vi "DAQ Manager.vi"(0 "DAQ Name":string="USB-6343", 1 "DAQ Mngr Action":T4, 9 "Value":dbl, 11 "error in (no error)":errorcluster) -> (3 "Vacuum Array":T1[](array[typedef]), 4 "device":tag, 6 "Pressure Array":T2[](array[typedef]), 8 "Plots":T3[](array[typedef]), 10 "Cart Sense":bool[](array[boolean]), 13 "Pressure Array":dbl[](array[numeric]), 14 "Connected":bool, 15 "error out":errorcluster)   [LabVIEW 2020]
uses:
  DAQ Mngr.ctl
  Main/Pressure Point.ctl
  Main/Pressure Output.ctl
  Main/Vacuum Output.ctl
  <vilib>/DAQmx/read.llb/DAQmx Read (Analog 2D DBL NChan NSamp).vi
  <vilib>/Analysis/baseanly.llb/Mean (DBL).vi
  <vilib>/DAQmx/write.llb/DAQmx Write (Digital 1D Bool 1Chan 1Samp).vi
  <vilib>/DAQmx/write.llb/DAQmx Write (Analog DBL 1Chan 1Samp).vi
  DAQ/DAQ Globals.vi
  <vilib>/DAQmx/miscellaneous.llb/DAQmx Fill In Error Info.vi
  <vilib>/DAQmx/create/channels.llb/DAQmx Create Channel (DO-Digital Output).vi
  <vilib>/DAQmx/create/channels.llb/DAQmx Create Channel (DI-Digital Input).vi
  <vilib>/DAQmx/create/channels.llb/DAQmx Create Channel (AO-Voltage-Basic).vi
  <vilib>/Analysis/NI_AALBase.lvlib
  Lib/Utilities.lvlib
panel:
  out "Vacuum Array":dbl[](array[numeric])
  in  "Buffer":u32=150
  out "PS Sense":bool
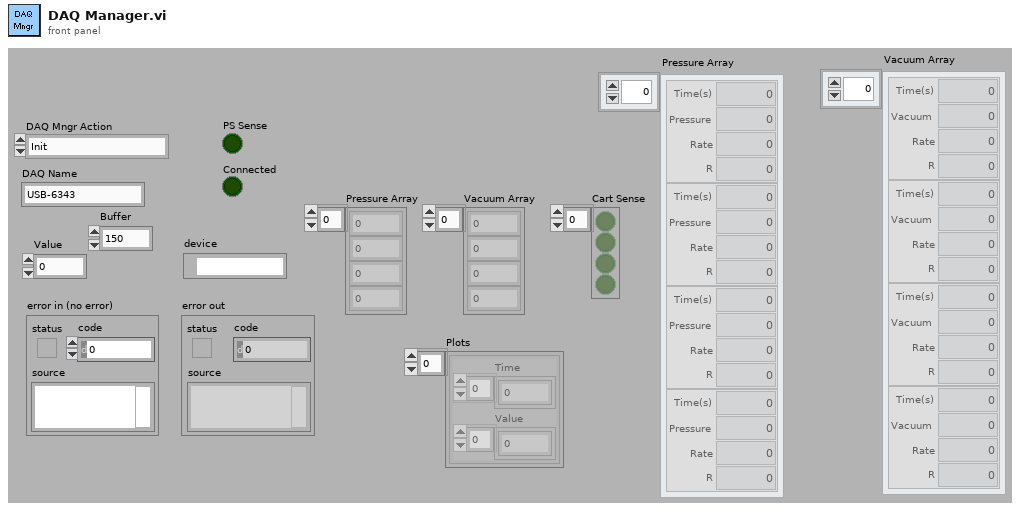
[diagram p1: front panel]
types:
  T1 = typedef "Vacuum Output.ctl" = cluster{"Time(s)":dbl, "Vacuum":dbl, "Rate":dbl, "R":dbl}
  T2 = typedef "Pressure Output.ctl" = cluster{"Time(s)":dbl, "Pressure":dbl, "Rate":dbl, "R":dbl}
  T3 = typedef "Pressure Point.ctl" = cluster{"Time":dbl[], "Value":dbl[]}
  T4 = typedef "DAQ Mngr.ctl" = enum16{"Init", "Read Pressure", "Read Vacuum", "Analyze Pressure", "Analyze Vacuum", "Read Cartridges", "Lock Cartridge", "Unlock Cartridge", "Read PS", "Pinch Valve Engage", "Pinch Valve Disengage", "Close"}
  T5 = cluster{"negative limit switch":bool, "positive limit switch":bool, "home switch":bool, "position marker":bool, "device enable":bool, "quick stop":bool, "general purpose J":bool, "general purpose I":bool, "general purpose H":bool, "general purpose G":bool, "general purpose F":bool, "general purpose E":bool, "general purpose D":bool, "general purpose C":bool, "general purpose B":bool, "general purpose A":bool}
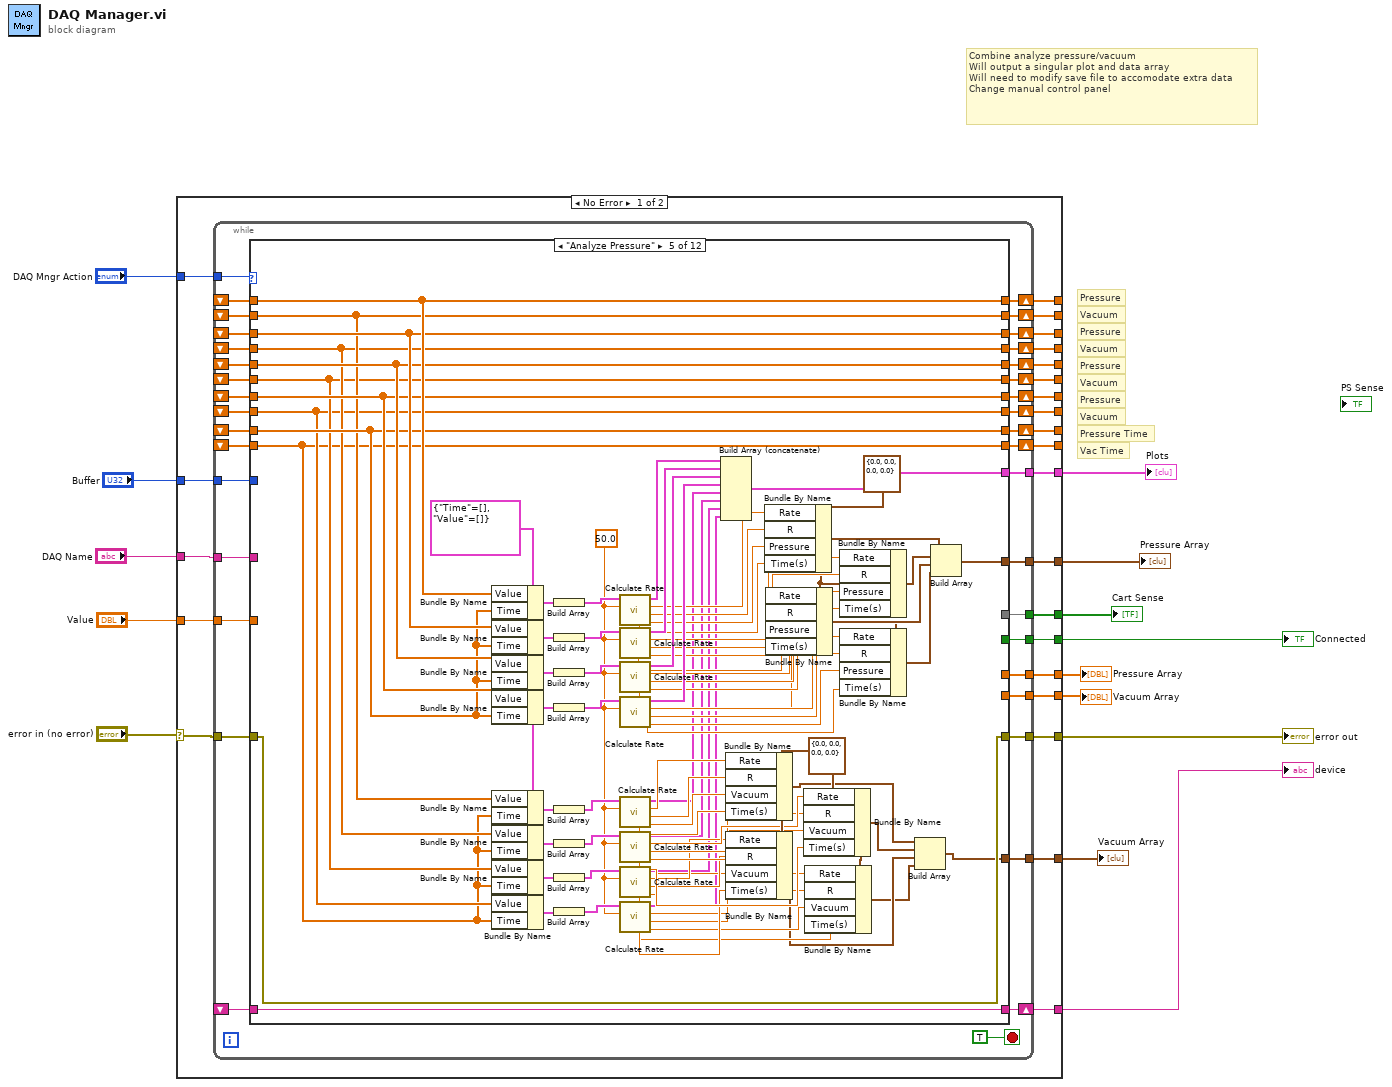
[diagram p0: block diagram]
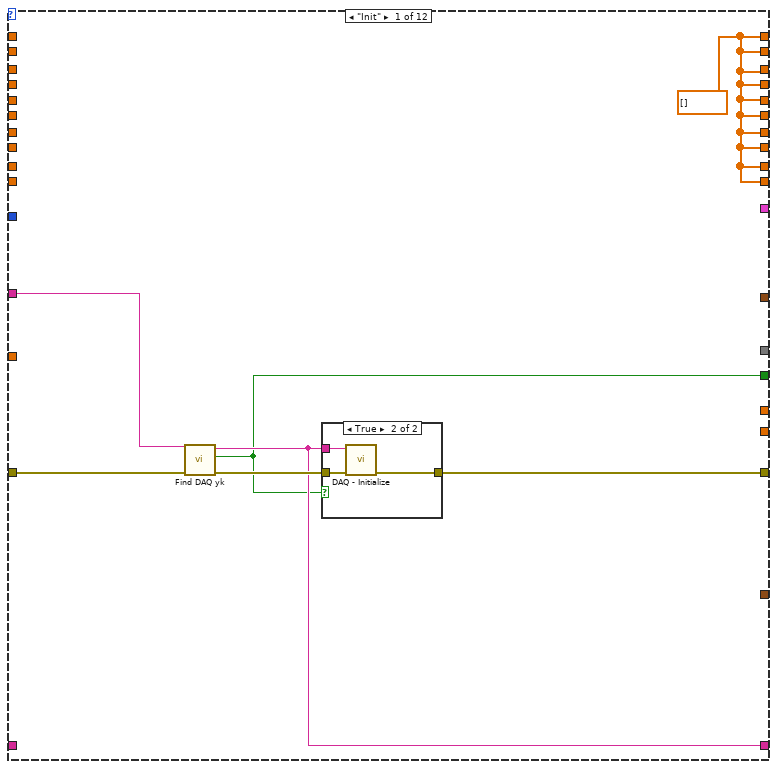
[diagram p2: hidden frame]
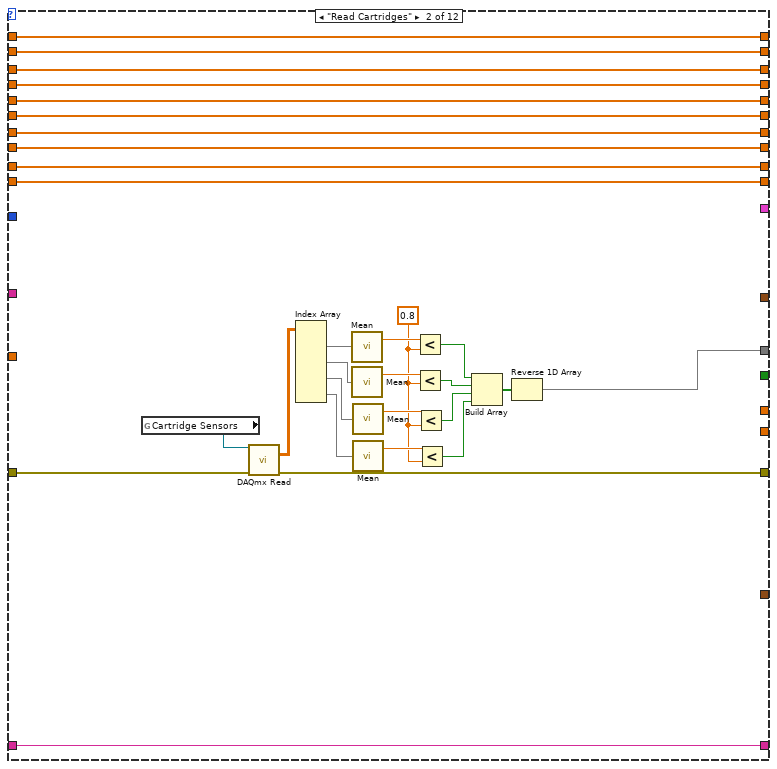
[diagram p4: hidden frame]
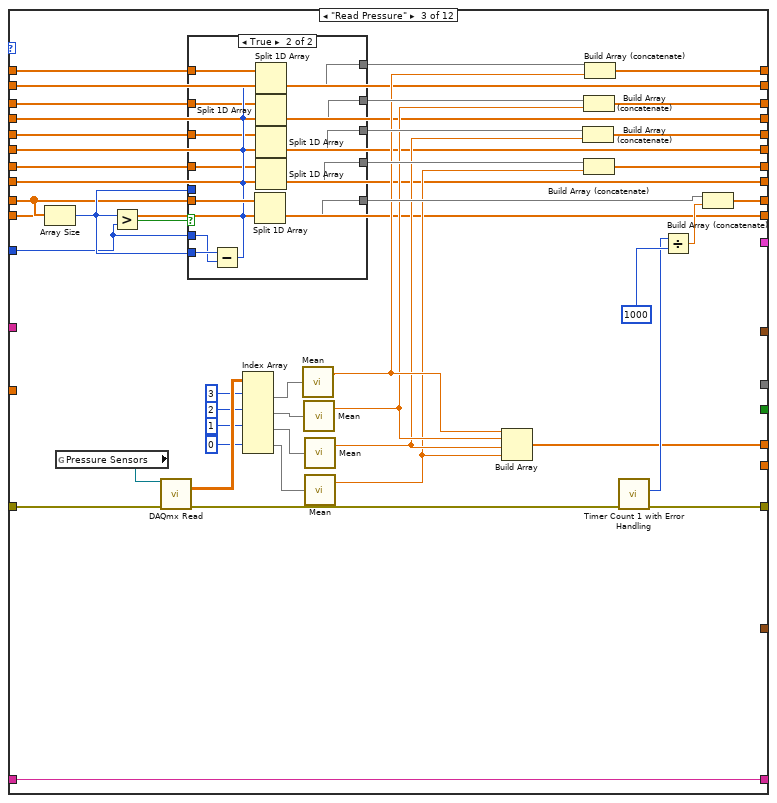
[diagram p5: hidden frame]
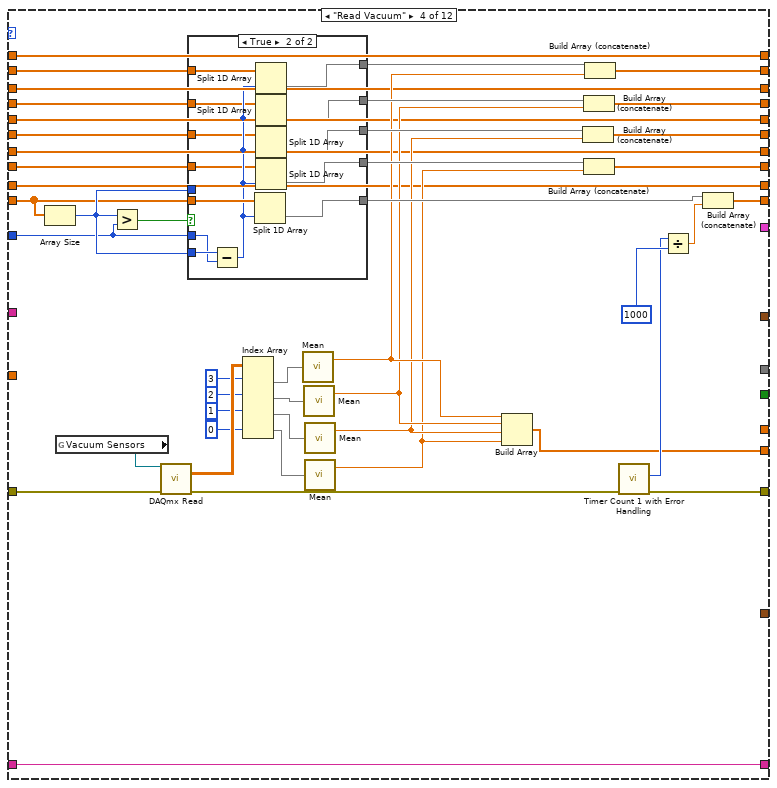
[diagram p7: hidden frame]
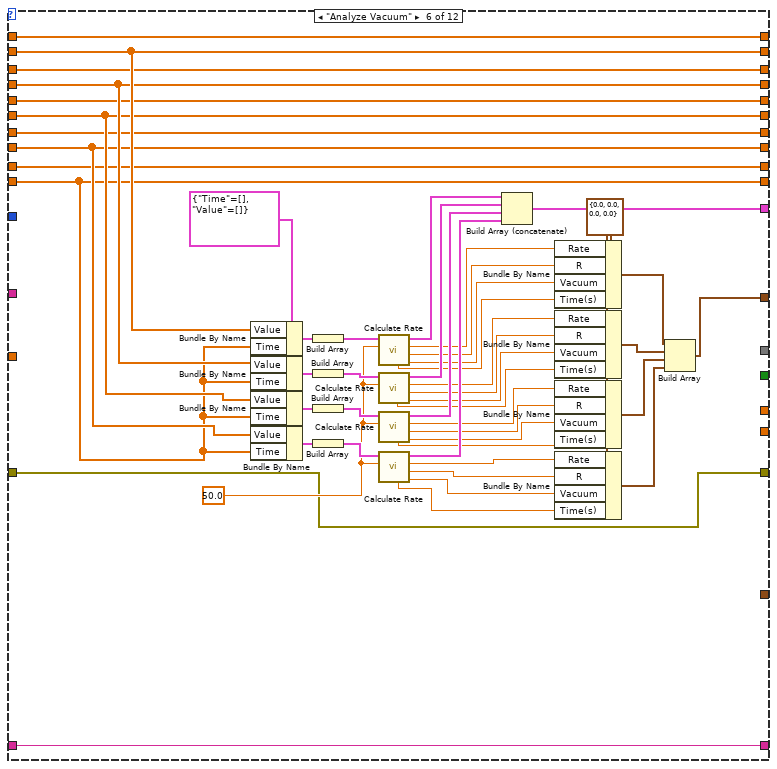
[diagram p9: hidden frame]
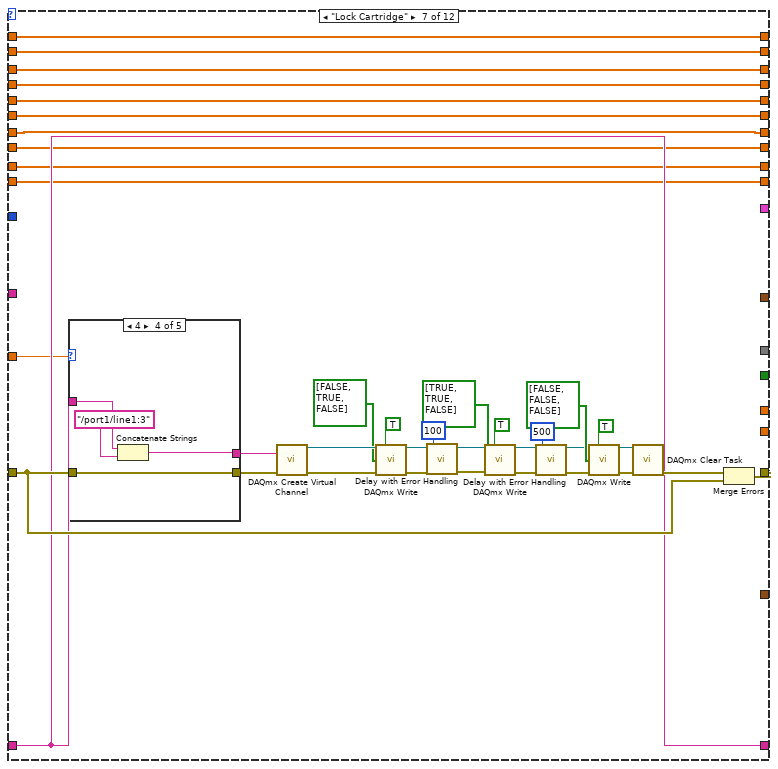
[diagram p10: hidden frame]
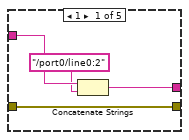
[diagram p11: hidden frame]
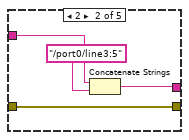
[diagram p12: hidden frame]
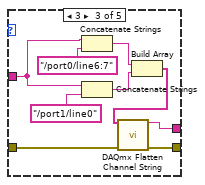
[diagram p13: hidden frame]
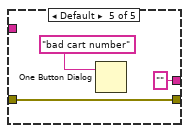
[diagram p14: hidden frame]
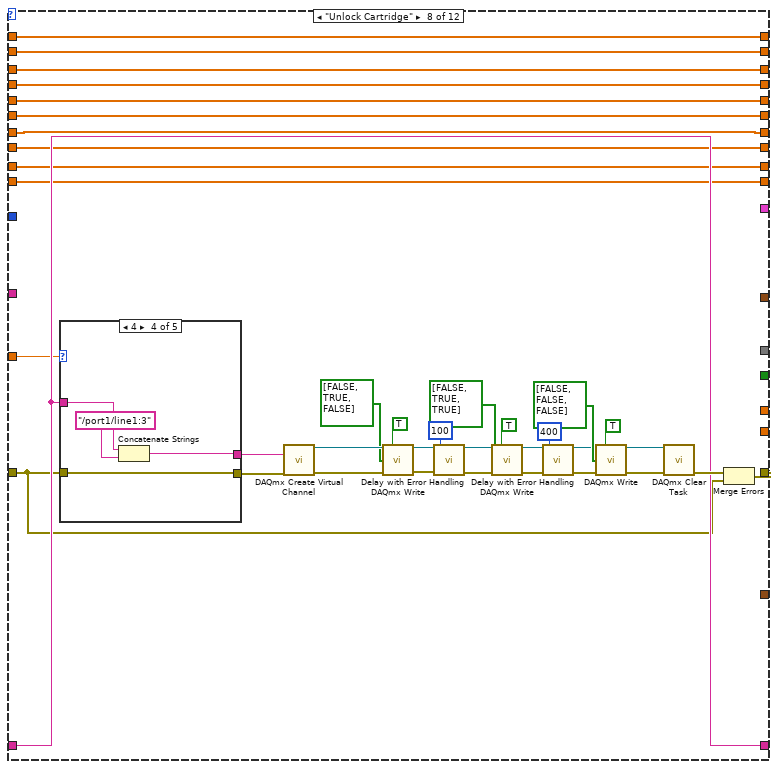
[diagram p15: hidden frame]
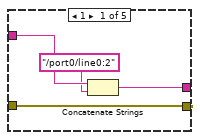
[diagram p16: hidden frame]
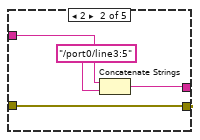
[diagram p17: hidden frame]
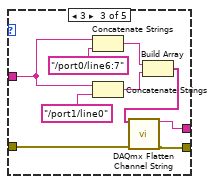
[diagram p18: hidden frame]
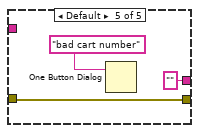
[diagram p19: hidden frame]
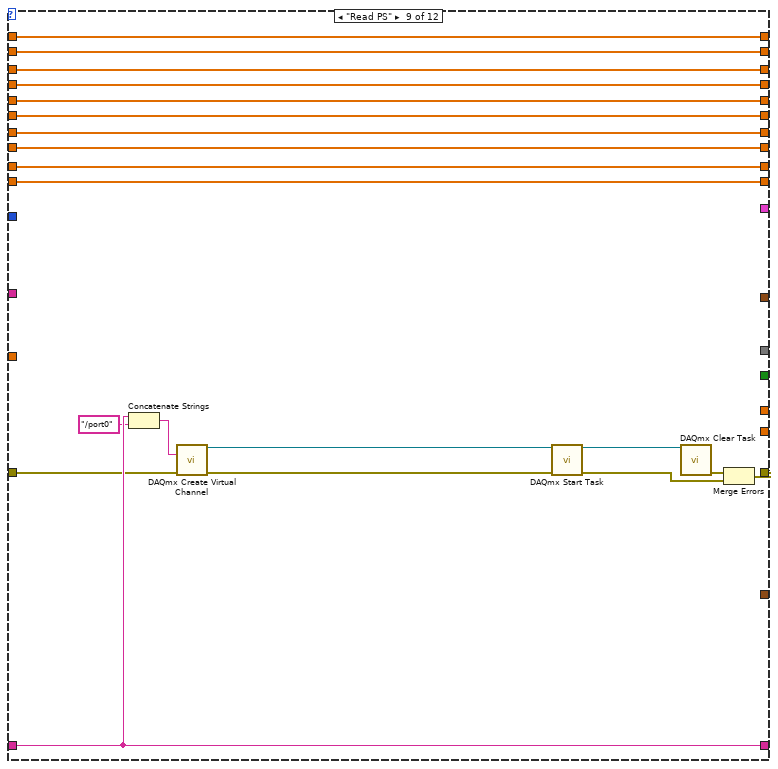
[diagram p20: hidden frame]
diagram:
  # "Vac Time"
  # "Pressure Time"
  # "Combine analyze pressure/vacuum\nWill output a singular plot and data array\nWill need to modify save file to accomodate extra data\nChange manual control panel"
  # "Vacuum"
  # "Pressure"
  # "Vacuum"
  # "Pressure"
  # "Vacuum"
  # "Pressure"
  # "Vacuum"
  # "Pressure"
  n1 = case shown="No Error" "error in (no error)" {
    selector: "error in (no error)" -> [w38 w616]
    tunnel: [w36 w616] -> w13
    tunnel: "DAQ Name" -> [w37 _]
    tunnel: "DAQ Mngr Action" -> [w35 _]
    tunnel: [w34 _] -> w10
    tunnel: [w33 _] -> w9
    tunnel: "Value" -> [w32 _]
    tunnel: [w31 _] -> w7
    tunnel: "Buffer" -> [w30 _]
    tunnel: [w29 _] -> _
    tunnel: [w28 _] -> _
    tunnel: [w27 _] -> _
    tunnel: [w26 _] -> _
    tunnel: [w25 _] -> _
    tunnel: [w24 _] -> w5
    tunnel: [w23 _] -> w3
    tunnel: [w22 _] -> w4
    tunnel: [w21 _] -> _
    tunnel: [w20 _] -> _
    tunnel: [w19 _] -> _
    tunnel: [w18 _] -> _
    tunnel: [w17 _] -> _
    tunnel: [w16 _] -> w2
    tunnel: [w15 _] -> w1
    frame No Error {
      n2 = while {
        tunnel: w38 -> [w72]
        tunnel: w37 -> [w71]
        tunnel: [w70] -> w36
        tunnel: w35 -> [w73]
        tunnel: [w69] -> w34
        tunnel: w32 -> [w67]
        shift-right: [w68] -> w33
        shift-left: _ -> [w66]
        tunnel: [w65] -> w31
        tunnel: w30 -> [w64]
        shift-right: [w63] -> w25
        shift-left: _ -> [w62]
        shift-right: [w61] -> w29
        shift-left: _ -> [w60]
        shift-right: [w59] -> w28
        shift-left: _ -> [w54]
        shift-right: [w58] -> w27
        shift-left: _ -> [w55]
        shift-right: [w57] -> w26
        shift-left: _ -> [w56]
        tunnel: [w53] -> w24
        tunnel: [w52] -> w23
        tunnel: [w51] -> w22
        shift-right: [w50] -> w21
        shift-left: _ -> [w45]
        shift-right: [w49] -> w20
        shift-left: _ -> [w44]
        shift-right: [w48] -> w19
        shift-left: _ -> [w43]
        shift-right: [w47] -> w18
        shift-left: _ -> [w42]
        shift-right: [w46] -> w17
        shift-left: _ -> [w41]
        tunnel: [w40] -> w16
        tunnel: [w39] -> w15
        stop <- TRUE stop-if-true
        n3 = case shown="\"Analyze Pressure\"" w73 {
          tunnel: w72 -> [w80 w114 w159 w222 w287 w340 w387 w464 w508 w551 w597 _]
          tunnel: w71 -> [w79 _ _ _ _ _ _ _ _ _ _ _]
          tunnel: [w78 w113 w142 w207 w287 w340 w407 w466 w509 w531 w577 w615] -> w70
          tunnel: [w76 _ _ _ _ _ _ _ _ _ _ _] -> w69
          tunnel: [w77 w115 w160 w223 w289 w343 w386 w465 w510 w519 w565 w609] -> w68
          tunnel: w67 -> [_ _ _ _ _ _ w385 w463 _ _ _ _]
          tunnel: w66 -> [_ w115 w160 w223 w289 w343 w386 w465 w510 w519 w565 w609]
          tunnel: [_ w96 _ _ _ _ _ _ _ _ _ _] -> w65
          tunnel: w64 -> [_ _ w145 w208 _ _ _ _ _ _ _ _]
          tunnel: [w75 w92 w144 w183 w321 w327 w380 w439 w498 w557 w603 w611] -> w63
          tunnel: w62 -> [_ w92 w143 w183 w321 w327 w380 w439 w498 w557 w603 w611]
          tunnel: [w75 w91 w140 w184 w320 w326 w379 w438 w497 w556 w602 w610] -> w61
          tunnel: w60 -> [_ w91 w139 w184 w320 w326 w379 w438 w497 w556 w602 w610]
          tunnel: [w75 w95 w138 w180 w324 w330 w383 w442 w501 w555 w601 w614] -> w59
          tunnel: [w75 w94 w137 w181 w323 w329 w382 w441 w500 w554 w600 w613] -> w58
          tunnel: [w75 w93 w136 w182 w322 w328 w381 w440 w499 w553 w599 w612] -> w57
          tunnel: w56 -> [_ w93 w135 w182 w322 w328 w381 w440 w499 w553 w599 w612]
          tunnel: w55 -> [_ w94 w134 w181 w323 w329 w382 w441 w500 w554 w600 w613]
          tunnel: w54 -> [_ w95 w133 w180 w324 w330 w383 w442 w501 w555 w601 w614]
          tunnel: [_ _ _ _ w319 w372 _ _ _ _ _ _] -> w53
          tunnel: [_ _ _ _ w291 w325 _ _ _ _ _ _] -> w52
          tunnel: [_ _ w125 _ _ _ _ _ _ _ _ _] -> w51
          tunnel: [w75 w90 w120 w194 w272 w336 w374 w437 w496 w516 w562 w608] -> w50
          tunnel: [w75 w89 w119 w193 w271 w335 w375 w436 w495 w515 w561 w607] -> w49
          tunnel: [w75 w88 w118 w192 w270 w334 w376 w435 w494 w514 w560 w606] -> w48
          tunnel: [w75 w87 w117 w191 w269 w333 w377 w434 w493 w513 w559 w605] -> w47
          tunnel: [w75 w86 w116 w190 w268 w332 w378 w433 w492 w512 w558 w604] -> w46
          tunnel: w45 -> [_ w90 w120 w189 w272 w336 w374 w437 w496 w516 w562 w608]
          tunnel: w44 -> [_ w89 w119 w188 w271 w335 w375 w436 w495 w515 w561 w607]
          tunnel: w43 -> [_ w88 w118 w187 w270 w334 w376 w435 w494 w514 w560 w606]
          tunnel: w42 -> [_ w87 w117 w186 w269 w333 w377 w434 w493 w513 w559 w605]
          tunnel: w41 -> [_ w86 w116 w185 w268 w332 w378 w433 w492 w512 w558 w604]
          tunnel: [_ _ _ w179 _ _ _ _ _ _ _ _] -> w40
          tunnel: [_ _ _ _ w246 _ _ _ _ _ _ _] -> w39
          frame "Init" {
            w75 = dbl[] []
            n4 = call "Find DAQ yk.vi"("error in"=w80, "DAQ Name"=w79) -> ("error out"=w81:errorcluster, "Device Found"=w76:bool, "device"=w77:tag)  [unwired: 5 in, 2 out]
            n5 = case shown="True" w76 {
              tunnel: w81 -> [w82 w85]
              tunnel: [w82 w84] -> w78
              tunnel: w77 -> [_ w83]
              frame False {
              }
              frame True {
                n6 = call "DAQ - Initialize.vi"("error in (no error)"=w85, "DAQ"=w83) -> ("error out"=w84:errorcluster)  [unwired: 9 in]
              }
            }
          }
          frame "Read Cartridges" {
            w102 = 0.8 ("y")
            n7 = global read "DAQ Globals.vi" "Cartridge Sensors"() -> (w112:refnum<k21>)
            n8 = call-poly <vilib>:"DAQmx Read.vi"("task/channels in"=w112, "error in"=w114) -> ("data"=w111:dbl[][], "error out"=w113:errorcluster)  [unwired: 11 in, 1 out]
            n9 = Index Array(array=w111) -> (element #1=w110:dbl[], element #2=w109:dbl[], element #3=w108:dbl[], element #4=w107:dbl[])  [unwired: 8 in]
            n10 = call-poly <vilib>:"Mean.vi"("X"=w110) -> ("mean"=w106:dbl)  [unwired: 1 out]
            n11 = call-poly <vilib>:"Mean.vi"("X"=w109) -> ("mean"=w105:dbl)  [unwired: 1 out]
            n12 = call-poly <vilib>:"Mean.vi"("X"=w108) -> ("mean"=w104:dbl)  [unwired: 1 out]
            n13 = call-poly <vilib>:"Mean.vi"("X"=w107) -> ("mean"=w103:dbl)  [unwired: 1 out]
            n14 = Less?(x=w106, y=w102) -> (x < y?=w101:bool)
            n15 = Less?(x=w105, y=w102) -> (x < y?=w100:bool)
            n16 = Less?(x=w104, y=w102) -> (x < y?=w99:bool)
            n17 = Less?(x=w103, y=w102) -> (x < y?=w98:bool)
            n18 = Build Array(w101, w100, w99, w98) -> (w97:bool[])
            n19 = Reverse 1D Array(array=w97) -> (reversed array=w96:bool[])
          }
          frame "Read Pressure" {
            n20 = Array Size(array=w139) -> (size(s)=w150:i32)
            n21 = global read "DAQ Globals.vi" "Pressure Sensors"() -> (w157:refnum<k21>)
            n22 = Greater?(x=w150, y=w145) -> (0:w151:bool)
            n23 = call-poly <vilib>:"DAQmx Read.vi"("task/channels in"=w157, "error in"=w159) -> ("data"=w156:dbl[][], "error out"=w158:errorcluster)  [unwired: 11 in, 1 out]
            n24 = case shown="True" w151 {
              tunnel: w143 -> [w165 w173]
              tunnel: w139 -> [w164 w178]
              tunnel: w145 -> [_ w176]
              tunnel: w150 -> [_ _]
              tunnel: w150 -> [_ w177]
              tunnel: [w165 w166] -> w149
              tunnel: [w164 w175] -> w148
              tunnel: w135 -> [w161 w172]
              tunnel: w134 -> [w162 w171]
              tunnel: w133 -> [w163 w170]
              tunnel: [w163 w169] -> w132
              tunnel: [w162 w168] -> w131
              tunnel: [w161 w167] -> w130
              frame False {
              }
              frame True {
                n25 = Subtract(x=w177, y=w176) -> (x-y=w174:u32)
                n26 = Split 1D Array(array=w178, index=w174) -> (second subarray=w175:dbl[])  [unwired: 1 out]
                n27 = Split 1D Array(array=w170, index=w174) -> (second subarray=w169:dbl[])  [unwired: 1 out]
                n28 = Split 1D Array(array=w171, index=w174) -> (second subarray=w168:dbl[])  [unwired: 1 out]
                n29 = Split 1D Array(array=w172, index=w174) -> (second subarray=w167:dbl[])  [unwired: 1 out]
                n30 = Split 1D Array(array=w173, index=w174) -> (second subarray=w166:dbl[])  [unwired: 1 out]
              }
            }
            n31 = Index Array(array=w156, index (row) #1=3 ("index (row)"), index (row) #2=2 ("index (row)"), index (row) #3=1 ("index (row)"), index (row) #4=0 ("index (row)")) -> (element #1=w155:dbl[], element #2=w154:dbl[], element #3=w153:dbl[], element #4=w152:dbl[])  [unwired: 4 in]
            n32 = call-poly <vilib>:"Mean.vi"("X"=w155) -> ("mean"=w124:dbl)  [unwired: 1 out]
            n33 = call-poly <vilib>:"Mean.vi"("X"=w154) -> ("mean"=w123:dbl)  [unwired: 1 out]
            n34 = call-poly <vilib>:"Mean.vi"("X"=w153) -> ("mean"=w122:dbl)  [unwired: 1 out]
            n35 = call-poly <vilib>:"Mean.vi"("X"=w152) -> ("mean"=w121:dbl)  [unwired: 1 out]
            n36 = Build Array(w124, w123, w122, w121) -> (w125:dbl[])
            n37 = Build Array (concatenate)(w130, w122) -> (w136:dbl[])
            n38 = Build Array (concatenate)(w131, w123) -> (w137:dbl[])
            n39 = Build Array (concatenate)(w149, w121) -> (w144:dbl[])
            n40 = Build Array (concatenate)(w132, w124) -> (w138:dbl[])
            n41 = call "Timer Count 1 with Error Handling.vi"("error in (no error)"=w158) -> ("error out"=w142:errorcluster, "Elapsed Time (ms)"=w141:u32)  [unwired: 7 in, 2 out]
            n42 = Divide(x=w141, y=u32 1000) -> (x/y=w147:dbl)
            n43 = Build Array (concatenate)(w148, w147) -> (w140:dbl[])
          }
          frame "Read Vacuum" {
            n44 = Array Size(array=w185) -> (size(s)=w213:i32)
            n45 = global read "DAQ Globals.vi" "Vacuum Sensors"() -> (w220:refnum<k21>)
            n46 = Greater?(x=w213, y=w208) -> (0:w214:bool)
            n47 = call-poly <vilib>:"DAQmx Read.vi"("task/channels in"=w220, "error in"=w222) -> ("data"=w219:dbl[][], "error out"=w221:errorcluster)  [unwired: 11 in, 1 out]
            n48 = case shown="True" w214 {
              tunnel: w186 -> [w228 w236]
              tunnel: w185 -> [w227 w241]
              tunnel: w208 -> [_ w239]
              tunnel: w213 -> [_ _]
              tunnel: w213 -> [_ w240]
              tunnel: [w228 w229] -> w212
              tunnel: [w227 w238] -> w211
              tunnel: w187 -> [w224 w235]
              tunnel: w188 -> [w225 w234]
              tunnel: w189 -> [w226 w233]
              tunnel: [w226 w232] -> w205
              tunnel: [w225 w231] -> w204
              tunnel: [w224 w230] -> w203
              frame False {
              }
              frame True {
                n49 = Subtract(x=w240, y=w239) -> (x-y=w237:u32)
                n50 = Split 1D Array(array=w241, index=w237) -> (second subarray=w238:dbl[])  [unwired: 1 out]
                n51 = Split 1D Array(array=w233, index=w237) -> (second subarray=w232:dbl[])  [unwired: 1 out]
                n52 = Split 1D Array(array=w234, index=w237) -> (second subarray=w231:dbl[])  [unwired: 1 out]
                n53 = Split 1D Array(array=w235, index=w237) -> (second subarray=w230:dbl[])  [unwired: 1 out]
                n54 = Split 1D Array(array=w236, index=w237) -> (second subarray=w229:dbl[])  [unwired: 1 out]
              }
            }
            n55 = Index Array(array=w219, index (row) #1=3 ("index (row)"), index (row) #2=2 ("index (row)"), index (row) #3=1 ("index (row)"), index (row) #4=0 ("index (row)")) -> (element #1=w218:dbl[], element #2=w217:dbl[], element #3=w216:dbl[], element #4=w215:dbl[])  [unwired: 4 in]
            n56 = call-poly <vilib>:"Mean.vi"("X"=w218) -> ("mean"=w198:dbl)  [unwired: 1 out]
            n57 = call-poly <vilib>:"Mean.vi"("X"=w217) -> ("mean"=w197:dbl)  [unwired: 1 out]
            n58 = call-poly <vilib>:"Mean.vi"("X"=w216) -> ("mean"=w196:dbl)  [unwired: 1 out]
            n59 = call-poly <vilib>:"Mean.vi"("X"=w215) -> ("mean"=w195:dbl)  [unwired: 1 out]
            n60 = Build Array(w198, w197, w196, w195) -> (w179:dbl[])
            n61 = Build Array (concatenate)(w203, w196) -> (w192:dbl[])
            n62 = Build Array (concatenate)(w204, w197) -> (w193:dbl[])
            n63 = Build Array (concatenate)(w212, w195) -> (w191:dbl[])
            n64 = Build Array (concatenate)(w205, w198) -> (w194:dbl[])
            n65 = call "Timer Count 1 with Error Handling.vi"("error in (no error)"=w221) -> ("error out"=w207:errorcluster, "Elapsed Time (ms)"=w206:u32)  [unwired: 7 in, 2 out]
            n66 = Divide(x=w206, y=u32 1000) -> (x/y=w210:dbl)
            n67 = Build Array (concatenate)(w211, w210) -> (w190:dbl[])
          }
          frame "Analyze Pressure" {
            w267 = T1 {"Time(s)"=0.0, "Vacuum"=0.0, "Rate"=0.0, "R"=0.0} ("Cluster")
            w283 = T2 {"Time(s)"=0.0, "Pressure"=0.0, "Rate"=0.0, "R"=0.0} ("Cluster")
            w273 = 50.0 ("Value")
            w282 = T3 {"Time"=[], "Value"=[]} ("output cluster")
            n68 = Bundle By Name(cluster=w282, "Value"=w324, "Time"=w320) -> (w318:T3)
            n69 = Bundle By Name(cluster=w282, "Value"=w323, "Time"=w320) -> (w317:T3)
            n70 = Bundle By Name(cluster=w282, "Value"=w322, "Time"=w320) -> (w315:T3)
            n71 = Bundle By Name(cluster=w282, "Value"=w321, "Time"=w320) -> (w313:T3)
            n72 = Bundle By Name(cluster=w282, "Value"=w272, "Time"=w268) -> (w278:T3)
            n73 = Bundle By Name(cluster=w282, "Value"=w271, "Time"=w268) -> (w279:T3)
            n74 = Bundle By Name(cluster=w282, "Value"=w270, "Time"=w268) -> (w280:T3)
            n75 = Bundle By Name(cluster=w282, "Value"=w269, "Time"=w268) -> (w281:T3)
            n76 = Build Array(w318) -> (w290:T3[])
            n77 = Build Array(w317) -> (w316:T3[])
            n78 = Build Array(w315) -> (w314:T3[])
            n79 = Build Array(w313) -> (w312:T3[])
            n80 = Build Array(w278) -> (w277:T3[])
            n81 = Build Array(w279) -> (w276:T3[])
            n82 = Build Array(w280) -> (w275:T3[])
            n83 = Build Array(w281) -> (w274:T3[])
            n84 = call "Calculate Rate.vi"("# of Pts"=w273, "Data In"=w290) -> ("Value"=w305:dbl, "residue"=w306:dbl, "slope"=w307:dbl, "Data Out"=w311:T3[], "Time"=w288:dbl)  [unwired: 5 in]
            n85 = call "Calculate Rate.vi"("# of Pts"=w273, "Data In"=w316) -> ("Value"=w302:dbl, "residue"=w303:dbl, "slope"=w304:dbl, "Data Out"=w310:T3[], "Time"=w286:dbl)  [unwired: 5 in]
            n86 = call "Calculate Rate.vi"("# of Pts"=w273, "Data In"=w314) -> ("Value"=w299:dbl, "residue"=w300:dbl, "slope"=w301:dbl, "Data Out"=w309:T3[], "Time"=w285:dbl)  [unwired: 5 in]
            n87 = call "Calculate Rate.vi"("# of Pts"=w273, "Data In"=w312) -> ("Value"=w296:dbl, "residue"=w297:dbl, "slope"=w298:dbl, "Data Out"=w308:T3[], "Time"=w284:dbl)  [unwired: 5 in]
            n88 = call "Calculate Rate.vi"("# of Pts"=w273, "Data In"=w277) -> ("Value"=w264:dbl, "residue"=w265:dbl, "slope"=w266:dbl, "Data Out"=w245:T3[], "Time"=w263:dbl)  [unwired: 5 in]
            n89 = call "Calculate Rate.vi"("# of Pts"=w273, "Data In"=w276) -> ("Value"=w260:dbl, "residue"=w261:dbl, "slope"=w262:dbl, "Data Out"=w244:T3[], "Time"=w259:dbl)  [unwired: 5 in]
            n90 = call "Calculate Rate.vi"("# of Pts"=w273, "Data In"=w275) -> ("Value"=w256:dbl, "residue"=w257:dbl, "slope"=w258:dbl, "Data Out"=w243:T3[], "Time"=w255:dbl)  [unwired: 5 in]
            n91 = call "Calculate Rate.vi"("# of Pts"=w273, "Data In"=w274) -> ("Value"=w252:dbl, "residue"=w253:dbl, "slope"=w254:dbl, "Data Out"=w242:T3[], "Time"=w251:dbl)  [unwired: 5 in]
            n92 = Build Array (concatenate)(w311, w310, w309, w308, w245, w244, w243, w242) -> (w319:T3[])
            n93 = Bundle By Name(cluster=w267, "Rate"=w266, "R"=w265, "Vacuum"=w264, "Time(s)"=w263) -> (w250:T1)
            n94 = Bundle By Name(cluster=w267, "Rate"=w258, "R"=w257, "Vacuum"=w256, "Time(s)"=w255) -> (w248:T1)
            n95 = Bundle By Name(cluster=w283, "Rate"=w307, "R"=w306, "Pressure"=w305, "Time(s)"=w288) -> (w295:T2)
            n96 = Bundle By Name(cluster=w283, "Rate"=w301, "R"=w300, "Pressure"=w299, "Time(s)"=w285) -> (w293:T2)
            n97 = Bundle By Name(cluster=w267, "Rate"=w262, "R"=w261, "Vacuum"=w260, "Time(s)"=w259) -> (w249:T1)
            n98 = Bundle By Name(cluster=w267, "Rate"=w254, "R"=w253, "Vacuum"=w252, "Time(s)"=w251) -> (w247:T1)
            n99 = Bundle By Name(cluster=w283, "Rate"=w304, "R"=w303, "Pressure"=w302, "Time(s)"=w286) -> (w294:T2)
            n100 = Bundle By Name(cluster=w283, "Rate"=w298, "R"=w297, "Pressure"=w296, "Time(s)"=w284) -> (w292:T2)
            n101 = Build Array(w250, w249, w248, w247) -> (w246:T1[])
            n102 = Build Array(w295, w294, w293, w292) -> (w291:T2[])
          }
          frame "Analyze Vacuum" {
            w331 = T1 {"Time(s)"=0.0, "Vacuum"=0.0, "Rate"=0.0, "R"=0.0} ("Cluster")
            w342 = 50.0 ("Value")
            w373 = T3 {"Time"=[], "Value"=[]} ("output cluster")
            n103 = Bundle By Name(cluster=w373, "Value"=w336, "Time"=w332) -> (w371:T3)
            n104 = Bundle By Name(cluster=w373, "Value"=w335, "Time"=w332) -> (w370:T3)
            n105 = Bundle By Name(cluster=w373, "Value"=w334, "Time"=w332) -> (w368:T3)
            n106 = Bundle By Name(cluster=w373, "Value"=w333, "Time"=w332) -> (w366:T3)
            n107 = Build Array(w371) -> (w344:T3[])
            n108 = Build Array(w370) -> (w369:T3[])
            n109 = Build Array(w368) -> (w367:T3[])
            n110 = Build Array(w366) -> (w365:T3[])
            n111 = call "Calculate Rate.vi"("# of Pts"=w342, "Data In"=w344) -> ("Value"=w358:dbl, "residue"=w359:dbl, "slope"=w360:dbl, "Data Out"=w364:T3[], "Time"=w341:dbl)  [unwired: 5 in]
            n112 = call "Calculate Rate.vi"("# of Pts"=w342, "Data In"=w369) -> ("Value"=w355:dbl, "residue"=w356:dbl, "slope"=w357:dbl, "Data Out"=w363:T3[], "Time"=w339:dbl)  [unwired: 5 in]
            n113 = call "Calculate Rate.vi"("# of Pts"=w342, "Data In"=w367) -> ("Value"=w352:dbl, "residue"=w353:dbl, "slope"=w354:dbl, "Data Out"=w362:T3[], "Time"=w338:dbl)  [unwired: 5 in]
            n114 = call "Calculate Rate.vi"("# of Pts"=w342, "Data In"=w365) -> ("Value"=w349:dbl, "residue"=w350:dbl, "slope"=w351:dbl, "Data Out"=w361:T3[], "Time"=w337:dbl)  [unwired: 5 in]
            n115 = Build Array (concatenate)(w364, w363, w362, w361) -> (w372:T3[])
            n116 = Bundle By Name(cluster=w331, "Rate"=w360, "R"=w359, "Vacuum"=w358, "Time(s)"=w341) -> (w348:T1)
            n117 = Bundle By Name(cluster=w331, "Rate"=w357, "R"=w356, "Vacuum"=w355, "Time(s)"=w339) -> (w347:T1)
            n118 = Bundle By Name(cluster=w331, "Rate"=w354, "R"=w353, "Vacuum"=w352, "Time(s)"=w338) -> (w346:T1)
            n119 = Bundle By Name(cluster=w331, "Rate"=w351, "R"=w350, "Vacuum"=w349, "Time(s)"=w337) -> (w345:T1)
            n120 = Build Array(w348, w347, w346, w345) -> (w325:T1[])
          }
          frame "Lock Cartridge" {
            n121 = case shown="4" w385 {
              tunnel: w386 -> [w411 w416 w424 w429 _]
              tunnel: w387 -> [w412 w414 w420 w427 w432]
              tunnel: [w412 w414 w419 w427 w432] -> w388
              tunnel: [w409 w413 w418 w426 ""] -> w384
              frame 1 {
                n122 = Concatenate Strings(w411, "/port0/line0:2" ("string")) -> (w409:string)
              }
              frame 2 {
                n123 = Concatenate Strings(w416, "/port0/line3:5" ("string")) -> (w413:string)
              }
              frame 3 {
                n124 = Concatenate Strings(w424, "/port0/line6:7" ("string")) -> (w422:string)
                n125 = Concatenate Strings(w424, "/port1/line0" ("string")) -> (w421:string)
                n126 = Build Array(w422, w421) -> (w417:string[])
                n127 = call <vilib>:"DAQmx Flatten Channel String.vi"("names in"=w417, "error in"=w420) -> ("names out"=w418:string, "error out"=w419:errorcluster)  [unwired: 12 in]
              }
              frame 4 {
                n128 = Concatenate Strings(w429, "/port1/line1:3" ("string")) -> (w426:string)
              }
              frame Default {
                n129 = One Button Dialog(message="bad cart number") -> ()  [unwired: 1 in, 1 out]
              }
            }
            n130 = call-poly <vilib>:"DAQmx Create Virtual Channel.vi"("lines"=w384, "error in"=w388) -> ("task out"=w403:refnum<k21>, "error out"=w404:errorcluster)  [unwired: 12 in]
            n131 = call-poly <vilib>:"DAQmx Write.vi"("task/channels in"=w403, "auto start"=TRUE, "data"=bool[] [FALSE, TRUE, FALSE], "error in"=w404) -> ("task out"=w395:refnum<k21>, "error out"=w400:errorcluster)  [unwired: 9 in, 1 out]
            n132 = call "Delay with Error Handling.vi"("error in (no error)"=w400, "Delay (ms)"=u32 100) -> ("error out"=w396:errorcluster)  [unwired: 9 in]
            n133 = call-poly <vilib>:"DAQmx Write.vi"("task/channels in"=w395, "auto start"=TRUE, "data"=bool[] [TRUE, TRUE, FALSE], "error in"=w396) -> ("task out"=w389:refnum<k21>, "error out"=w391:errorcluster)  [unwired: 9 in, 1 out]
            n134 = call "Delay with Error Handling.vi"("error in (no error)"=w391, "Delay (ms)"=u32 500) -> ("error out"=w390:errorcluster)  [unwired: 9 in]
            n135 = call-poly <vilib>:"DAQmx Write.vi"("task/channels in"=w389, "auto start"=TRUE, "data"=bool[] [FALSE, FALSE, FALSE], "error in"=w390) -> ("task out"=w406:refnum<k21>, "error out"=w405:errorcluster)  [unwired: 9 in, 1 out]
            n136 = call <vilib>:"DAQmx Clear Task.vi"("task in"=w406, "error in"=w405) -> ("error out"=w408:errorcluster)  [unwired: 13 in]
            n137 = Merge Errors(w408, w387) -> (w407:errorcluster)
          }
          frame "Unlock Cartridge" {
            n138 = case shown="4" w463 {
              tunnel: w465 -> [w470 w475 w476 w488 _]
              tunnel: w464 -> [w471 w473 w479 w486 w491]
              tunnel: [w471 w473 w478 w486 w491] -> w443
              tunnel: [w468 w472 w477 w485 ""] -> w444
              frame 1 {
                n139 = Concatenate Strings(w470, "/port0/line0:2" ("string")) -> (w468:string)
              }
              frame 2 {
                n140 = Concatenate Strings(w475, "/port0/line3:5" ("string")) -> (w472:string)
              }
              frame 3 {
                n141 = Concatenate Strings(w476, "/port0/line6:7" ("string")) -> (w482:string)
                n142 = Concatenate Strings(w476, "/port1/line0" ("string")) -> (w481:string)
                n143 = Build Array(w482, w481) -> (w480:string[])
                n144 = call <vilib>:"DAQmx Flatten Channel String.vi"("names in"=w480, "error in"=w479) -> ("names out"=w477:string, "error out"=w478:errorcluster)  [unwired: 12 in]
              }
              frame 4 {
                n145 = Concatenate Strings(w488, "/port1/line1:3" ("string")) -> (w485:string)
              }
              frame Default {
                n146 = One Button Dialog(message="bad cart number") -> ()  [unwired: 1 in, 1 out]
              }
            }
            n147 = call-poly <vilib>:"DAQmx Create Virtual Channel.vi"("lines"=w444, "error in"=w443) -> ("task out"=w461:refnum<k21>, "error out"=w462:errorcluster)  [unwired: 12 in]
            n148 = call-poly <vilib>:"DAQmx Write.vi"("task/channels in"=w461, "auto start"=TRUE, "data"=bool[] [FALSE, TRUE, FALSE], "error in"=w462) -> ("task out"=w453:refnum<k21>, "error out"=w458:errorcluster)  [unwired: 9 in, 1 out]
            n149 = call "Delay with Error Handling.vi"("error in (no error)"=w458, "Delay (ms)"=u32 100) -> ("error out"=w454:errorcluster)  [unwired: 9 in]
            n150 = call-poly <vilib>:"DAQmx Write.vi"("task/channels in"=w453, "auto start"=TRUE, "data"=bool[] [FALSE, TRUE, TRUE], "error in"=w454) -> ("task out"=w447:refnum<k21>, "error out"=w449:errorcluster)  [unwired: 9 in, 1 out]
            n151 = call "Delay with Error Handling.vi"("error in (no error)"=w449, "Delay (ms)"=u32 400) -> ("error out"=w448:errorcluster)  [unwired: 9 in]
            n152 = call-poly <vilib>:"DAQmx Write.vi"("task/channels in"=w447, "auto start"=TRUE, "data"=bool[] [FALSE, FALSE, FALSE], "error in"=w448) -> ("task out"=w446:refnum<k21>, "error out"=w445:errorcluster)  [unwired: 9 in, 1 out]
            n153 = call <vilib>:"DAQmx Clear Task.vi"("task in"=w446, "error in"=w445) -> ("error out"=w467:errorcluster)  [unwired: 13 in]
            n154 = Merge Errors(w467, w464) -> (w466:errorcluster)
          }
          frame "Read PS" {
            n155 = Concatenate Strings(w510, "/port0" ("string")) -> (w507:string)
            n156 = call-poly <vilib>:"DAQmx Create Virtual Channel.vi"("lines"=w507, "error in"=w508) -> ("task out"=w505:refnum<k21>, "error out"=w504:errorcluster)  [unwired: 12 in]
            n157 = call <vilib>:"DAQmx Start Task.vi"("task/channels in"=w505, "error in"=w504) -> ("task out"=w503:refnum<k21>, "error out"=w502:errorcluster)  [unwired: 12 in]
            n158 = call <vilib>:"DAQmx Clear Task.vi"("task in"=w503) -> ("error out"=w511:errorcluster)  [unwired: 14 in]
            n159 = Merge Errors(w511, w502) -> (w509:errorcluster)
          }
          frame "Pinch Valve Engage" {
            n160 = Concatenate Strings(w519, "/ao1" ("string")) -> (w522:string)
            n161 = call-poly <vilib>:"DAQmx Create Virtual Channel.vi"("maximum value"=5.0, "minimum value"=0.0, "physical channels"=w522, "error in"=w551) -> ("task out"=w549:refnum<k21>, "error out"=w550:errorcluster)  [unwired: 10 in]
            n162 = call-poly <vilib>:"DAQmx Write.vi"("task/channels in"=w549, "data"=0.0, "error in"=w550) -> ("task out"=w546:refnum<k21>, "error out"=w529:errorcluster)  [unwired: 10 in, 1 out]
            n163 = call "Delay with Error Handling.vi"("error in (no error)"=w529, "Delay (ms)"=u32 500) -> ("error out"=w528:errorcluster)  [unwired: 9 in]
            n164 = Concatenate Strings(w519, "/ao0" ("string")) -> (w520:string)
            n165 = call <vilib>:"DAQmx Clear Task.vi"("task in"=w546, "error in"=w528) -> ("error out"=w539:errorcluster)  [unwired: 13 in]
            n166 = call-poly <vilib>:"DAQmx Create Virtual Channel.vi"("maximum value"=5.0, "minimum value"=0.0, "physical channels"=w520, "error in"=w539) -> ("task out"=w543:refnum<k21>, "error out"=w544:errorcluster)  [unwired: 10 in]
            n167 = call-poly <vilib>:"DAQmx Write.vi"("task/channels in"=w543, "data"=5.0, "error in"=w544) -> ("task out"=w540:refnum<k21>, "error out"=w526:errorcluster)  [unwired: 10 in, 1 out]
            n168 = call "Delay with Error Handling.vi"("error in (no error)"=w526, "Delay (ms)"=u32 500) -> ("error out"=w525:errorcluster)  [unwired: 9 in]
            n169 = Concatenate Strings(w519, "/ao0" ("string")) -> (w517:string)
            n170 = call <vilib>:"DAQmx Clear Task.vi"("task in"=w540, "error in"=w525) -> ("error out"=w530:errorcluster)  [unwired: 13 in]
            n171 = call-poly <vilib>:"DAQmx Create Virtual Channel.vi"("maximum value"=5.0, "minimum value"=0.0, "physical channels"=w517, "error in"=w530) -> ("task out"=w536:refnum<k21>, "error out"=w537:errorcluster)  [unwired: 10 in]
            n172 = call-poly <vilib>:"DAQmx Write.vi"("task/channels in"=w536, "data"=0.0, "error in"=w537) -> ("task out"=w533:refnum<k21>, "error out"=w532:errorcluster)  [unwired: 10 in, 1 out]
            n173 = call <vilib>:"DAQmx Clear Task.vi"("task in"=w533, "error in"=w532) -> ("error out"=w531:errorcluster)  [unwired: 13 in]
          }
          frame "Pinch Valve Disengage" {
            n174 = Concatenate Strings(w565, "/ao1" ("string")) -> (w569:string)
            n175 = call-poly <vilib>:"DAQmx Create Virtual Channel.vi"("maximum value"=5.0, "minimum value"=0.0, "physical channels"=w569, "error in"=w597) -> ("task out"=w595:refnum<k21>, "error out"=w596:errorcluster)  [unwired: 10 in]
            n176 = call-poly <vilib>:"DAQmx Write.vi"("task/channels in"=w595, "data"=5.0, "error in"=w596) -> ("task out"=w592:refnum<k21>, "error out"=w575:errorcluster)  [unwired: 10 in, 1 out]
            n177 = call "Delay with Error Handling.vi"("error in (no error)"=w575, "Delay (ms)"=u32 500) -> ("error out"=w574:errorcluster)  [unwired: 9 in]
            n178 = Concatenate Strings(w565, "/ao0" ("string")) -> (w566:string)
            n179 = call <vilib>:"DAQmx Clear Task.vi"("task in"=w592, "error in"=w574) -> ("error out"=w585:errorcluster)  [unwired: 13 in]
            n180 = call-poly <vilib>:"DAQmx Create Virtual Channel.vi"("maximum value"=5.0, "minimum value"=0.0, "physical channels"=w566, "error in"=w585) -> ("task out"=w589:refnum<k21>, "error out"=w590:errorcluster)  [unwired: 10 in]
            n181 = call-poly <vilib>:"DAQmx Write.vi"("task/channels in"=w589, "data"=5.0, "error in"=w590) -> ("task out"=w586:refnum<k21>, "error out"=w572:errorcluster)  [unwired: 10 in, 1 out]
            n182 = call "Delay with Error Handling.vi"("error in (no error)"=w572, "Delay (ms)"=u32 500) -> ("error out"=w571:errorcluster)  [unwired: 9 in]
            n183 = Concatenate Strings(w565, "/ao0" ("string")) -> (w563:string)
            n184 = call <vilib>:"DAQmx Clear Task.vi"("task in"=w586, "error in"=w571) -> ("error out"=w576:errorcluster)  [unwired: 13 in]
            n185 = call-poly <vilib>:"DAQmx Create Virtual Channel.vi"("maximum value"=5.0, "minimum value"=0.0, "physical channels"=w563, "error in"=w576) -> ("task out"=w582:refnum<k21>, "error out"=w583:errorcluster)  [unwired: 10 in]
            n186 = call-poly <vilib>:"DAQmx Write.vi"("task/channels in"=w582, "data"=0.0, "error in"=w583) -> ("task out"=w579:refnum<k21>, "error out"=w578:errorcluster)  [unwired: 10 in, 1 out]
            n187 = call <vilib>:"DAQmx Clear Task.vi"("task in"=w579, "error in"=w578) -> ("error out"=w577:errorcluster)  [unwired: 13 in]
          }
          frame "Close" {
            n188 = call "DAQ - Close.vi"() -> ("error out"=w615:errorcluster)  [unwired: 11 in]
          }
        }
      }
    }
    frame Error {
      (unwired) T5 {"negative limit switch"=FALSE, "positive limit switch"=FALSE, "home switch"=FALSE, "position marker"=FALSE, "device enable"=FALSE, "quick stop"=FALSE, "general purpose J"=FALSE, "general purpose I"=FALSE, "general purpose H"=FALSE, "general purpose G"=FALSE, "general purpose F"=FALSE, "general purpose E"=FALSE, "general purpose D"=FALSE, "general purpose C"=FALSE, "general purpose B"=FALSE, "general purpose A"=FALSE} ("digital inputs")
    }
  }
  "error out" <- w13
  "Connected" <- w10
  "device" <- w9
  "Cart Sense" <- w7
  "Plots" <- w5
  "Pressure Array" <- w3
  "Pressure Array" <- w4
  "Vacuum Array" <- w1
  "Vacuum Array" <- w2
